vi "IVA Vision FPGA (Host).vi"() -> ()   [LabVIEW 2015]
uses:
  <vilib>/visionFPGA/Controls/IMAQ FPGA Image Size.ctl
  <vilib>/FPGAPlugInAG/cRIO-9030/niLvFpga_Open_cRIO-9030.vi
  <vilib>/rvi/interface/common/dynamic/niFpgaDynamicAddResources.vi
  <vilib>/FPGAPlugInAG/Dynamic/niLvFpga_Download_Dynamic.vi
  <vilib>/FPGAPlugInAG/Dynamic/niLvFpga_Run_Dynamic.vi
  <vilib>/visionFPGA/Basics/Configure Image Transfer from Target/IMAQ FPGA Configure Image Transfer from Target U8.vi
  <vilib>/visionFPGA/Basics/Image Transfer from Target/IMAQ FPGA Image Transfer from Target U8.vi
  <vilib>/visionFPGA/Basics/Configure Image Transfer to Target/IMAQ FPGA Configure Image Transfer to Target U32.vi
  <vilib>/visionFPGA/Basics/Image Transfer to Target/IMAQ FPGA Image Transfer to Target U32.vi
  <vilib>/FPGAPlugInAG/Dynamic/niLvFpga_Close_Dynamic.vi
  <vilib>/rvi/interface/nirviOpenFPGA/nirviOpenFPGA.xnode
  FPGA Bitfiles/IVAVisionFPGA.lvbitx
  IVA Vision FPGA (FPGA).vi
  <vilib>/rvi/interface/nirviMethod/nirviMethod.xnode
  <vilib>/rvi/interface/nirviCloseFPGA/nirviCloseFPGA.xnode
  <vilib>/visionFPGA/NI_VDM_FPGA_Basics.lvlib
panel:
  out "Image Out":T1(plugin-control)
  out "Error Out":errorcluster
  out "Image":T1(plugin-control)
  in  "Stop":bool
  in  "Image File Path":path
  # "Overview: Demonstrates how to use IMAQ FPGA Image Transfer Host to Target to transfer an image to a FPGA target for processing.\nRequirements:\n- LabVIEW FPGA\n- Vision Development Software\nInstructions:\n1. Select an Image File Path\n2. Run the VI."
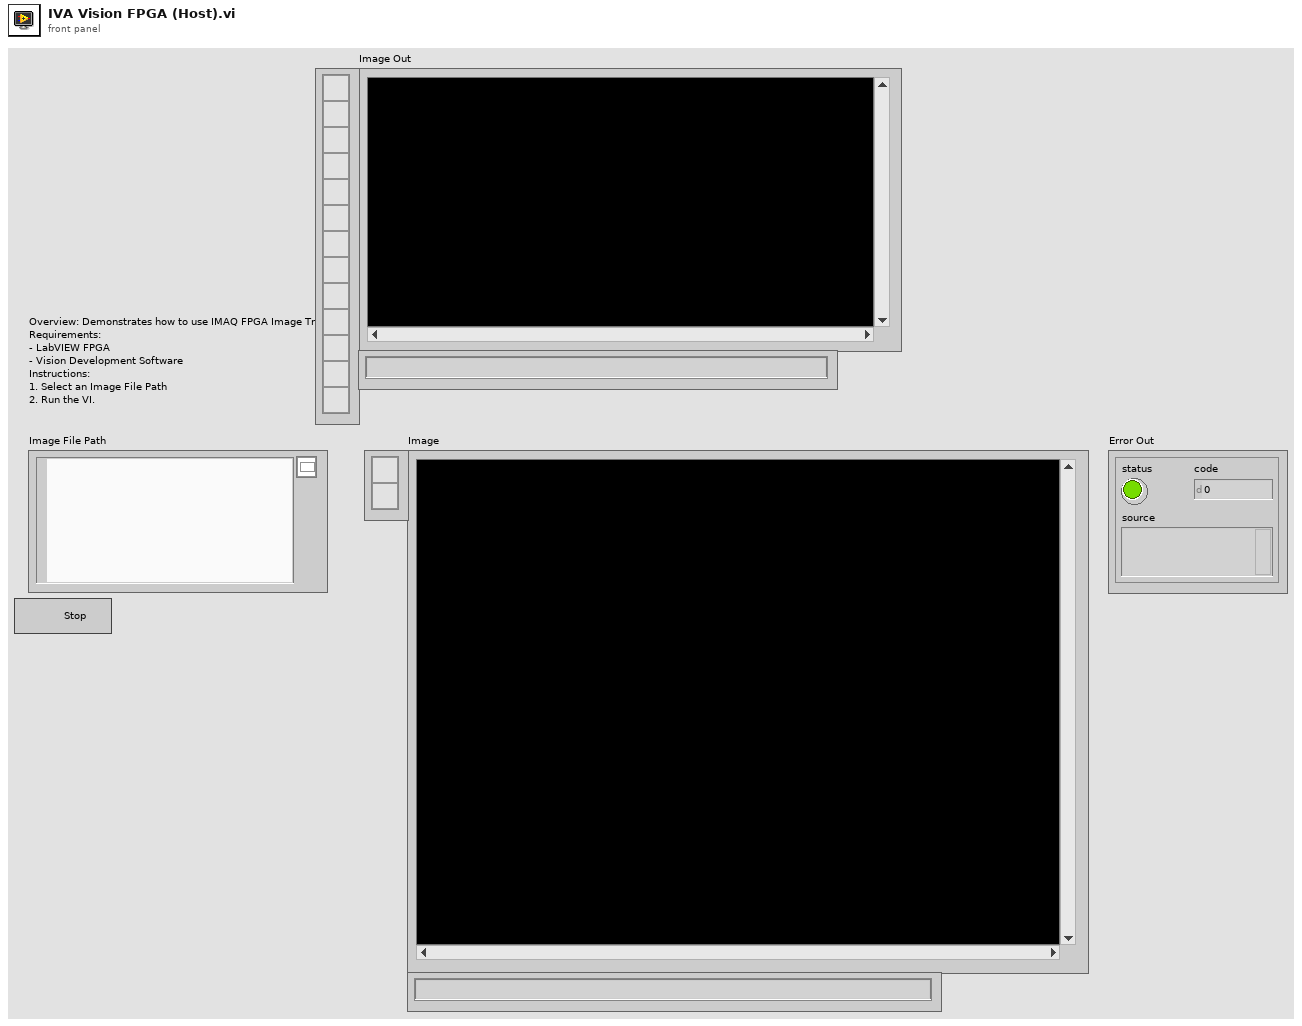
[diagram p1: front panel]
types:
  T1 = typedef "IMAQ Image.ctl" = refnum<image>
  T2 = typedef "IMAQ FPGA Image Size.ctl" = cluster{"Width":u32, "Height":u32}
  T3 = typedef "Image Type" = u32
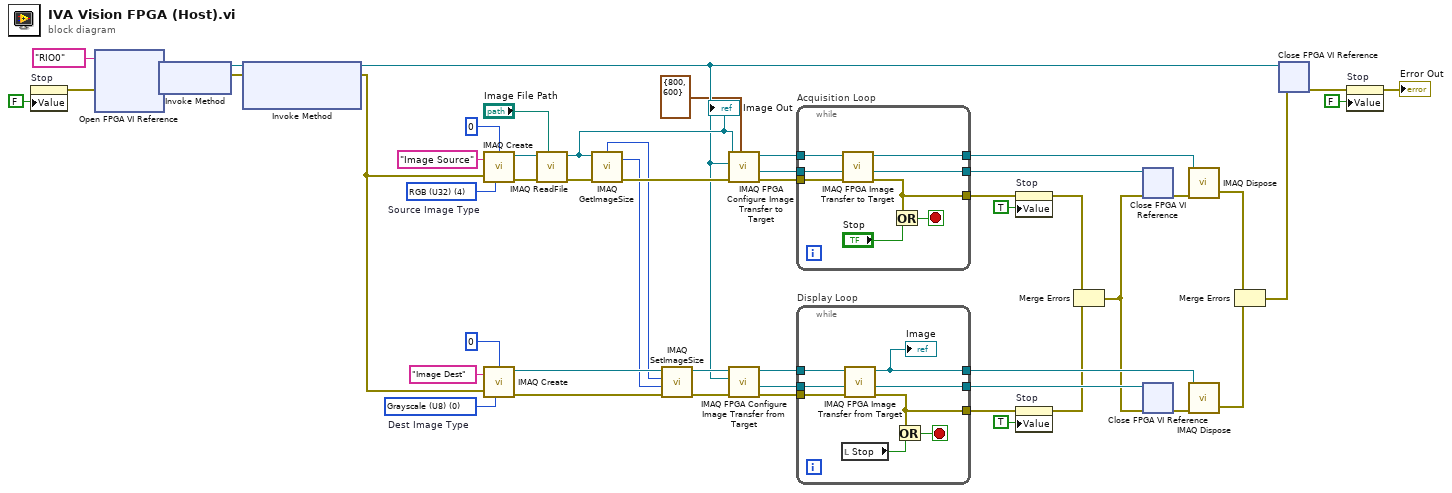
[diagram p0: block diagram]
diagram:
  w16 = T3 0 items=["Grayscale (U8)", "Grayscale (I16)", "Grayscale (SGL)", "Complex (CSG)", "RGB (U32)", "HSL (U32)", "RGB (U64)", "Grayscale (U16)"]  # Dest Image Type
  w17 = T3 4 items=["Grayscale (U8)", "Grayscale (I16)", "Grayscale (SGL)", "Complex (CSG)", "RGB (U32)", "HSL (U32)", "RGB (U64)", "Grayscale (U16)"]  # Source Image Type
  n1 = property on="Stop" class="Bool (strict)"("Value"=FALSE ("Stop")) -> (error out=w44:errorcluster)  [unwired: 2 in, 1 out]
  n2 = xnode "Open FPGA VI Reference"("error in"=w44, "resource name"=tag "RIO0") -> ("FPGA VI Reference Out"=w39:refnum<k20>, "error out"=w41:errorcluster)
  n3 = xnode "Invoke Method"("FPGA VI Reference In"=w39, "error in"=w41) -> ("FPGA VI Reference Out"=w43:refnum<k20>, "error out"=w42:errorcluster)
  n4 = xnode "Invoke Method"("FPGA VI Reference In"=w43, "error in"=w42) -> ("FPGA VI Reference Out"=w13:refnum<k20>, "error out"=w40:errorcluster)  [unwired: 1 in]
  n5 = call "IMAQ Create"("Border Size"=0, "Image Name"="Image Source", "Image Type"=w17, "error in (no error)"=w40) -> ("New Image"=w52:T1, "error out"=w51:errorcluster)  [unwired: 1 in]
  n6 = call "IMAQ Create"("Border Size"=0, "Image Name"="Image Dest", "Image Type"=w16, "error in (no error)"=w40) -> ("New Image"=w46:T1, "error out"=w14:errorcluster)  [unwired: 1 in]
  n7 = call "IMAQ ReadFile"("File Path"="Image File Path", "error in (no error)"=w51, "Image"=w52) -> ("error out"=w47:errorcluster, "Image Out"=w37:T1)  [unwired: 4 in, 3 out]
  "Image Out" <- w37
  n8 = call "IMAQ GetImageSize"("Image"=w37, "error in (no error)"=w47) -> ("Y Resolution"=w21:i32, "X Resolution"=w20:i32, "error out"=w38:errorcluster)  [unwired: 2 in]
  n9 = call "IMAQ SetImageSize"("error in (no error)"=w14, "Y Resolution"=w21, "X Resolution"=w20, "Image"=w46) -> ("error out"=w32:errorcluster, "Image Out"=w33:T1)  [unwired: 1 in]
  n10 = call-poly <vilib>:"IMAQ FPGA Configure Image Transfer to Target.vi"("Image Size"=T2 {"Width"=800, "Height"=600}, "error in (no error)"=w38, "FPGA VI Reference In"=w13, "Image"=w37) -> ("error out"=w34:errorcluster, "DMA FIFO Reference Out"=w35:refnum<k20>, "Image Out"=w36:T1)  [unwired: 4 in, 1 out]
  n11 = call-poly <vilib>:"IMAQ FPGA Configure Image Transfer from Target.vi"("error in (no error)"=w32, "FPGA VI Reference In"=w13, "Image"=w33) -> ("error out"=w30:errorcluster, "DMA FIFO Reference Out"=w29:refnum<k20>, "Image Out"=w31:T1)  [unwired: 6 in]
  n12 = while "Acquisition Loop" {
    tunnel: [w54] -> w12
    tunnel: w36 -> [w59]
    tunnel: w35 -> [w58]
    tunnel: w34 -> [w57]
    tunnel: [w56] -> w6
    tunnel: [w55] -> w28
    stop <- w60 stop-if-true
    n13 = call-poly <vilib>:"IMAQ FPGA Image Transfer to Target.vi"("error in (no error)"=w57, "DMA FIFO Reference In"=w58, "Image"=w59) -> ("error out"=w54:errorcluster, "DMA FIFO Reference Out"=w56:refnum<k20>, "Image Out"=w55:T1)  [unwired: 6 in]
    n14 = Or(x=w54, y="Stop") -> (x .or. y?=w60:bool)
  }
  n15 = while "Display Loop" {
    tunnel: w31 -> [w68]
    tunnel: [w66] -> w25
    tunnel: w30 -> [w65]
    tunnel: w29 -> [w64]
    tunnel: [w63] -> w26
    tunnel: [w62] -> w9
    stop <- w69 stop-if-true
    n16 = local read "Stop"() -> (w67:bool)
    n17 = call-poly <vilib>:"IMAQ FPGA Image Transfer from Target.vi"("error in (no error)"=w65, "DMA FIFO Reference In"=w64, "Image"=w68) -> ("error out"=w62:errorcluster, "DMA FIFO Reference Out"=w63:refnum<k20>, "Image Out"=w66:T1)  [unwired: 6 in]
    "Image" <- w66
    n18 = Or(x=w62, y=w67) -> (x .or. y?=w69:bool)
  }
  n19 = property on="Stop" class="Bool (strict)"(error in=w12, "Value"=TRUE ("Stop")) -> (error out=w8:errorcluster)  [unwired: 1 in, 1 out]
  n20 = property on="Stop" class="Bool (strict)"(error in=w9, "Value"=TRUE ("Stop")) -> (error out=w7:errorcluster)  [unwired: 1 in, 1 out]
  n21 = Merge Errors(w8, w7) -> (w5:errorcluster)
  n22 = xnode "Close FPGA VI Reference"("FPGA VI Reference In"=w6, "error in"=w5) -> ("error out"=w27:errorcluster)
  n23 = xnode "Close FPGA VI Reference"("FPGA VI Reference In"=w26, "error in"=w5) -> ("error out"=w24:errorcluster)
  n24 = call "IMAQ Dispose"("Image"=w28, "error in (no error)"=w27) -> ("error out"=w22:errorcluster)  [unwired: 4 in]
  n25 = call "IMAQ Dispose"("Image"=w25, "error in (no error)"=w24) -> ("error out"=w23:errorcluster)  [unwired: 4 in]
  n26 = Merge Errors(w22, w23) -> (w15:errorcluster)
  n27 = xnode "Close FPGA VI Reference"("FPGA VI Reference In"=w13, "error in"=w15) -> ("error out"=w3:errorcluster)
  n28 = property on="Stop" class="Bool (strict)"(error in=w3, "Value"=FALSE ("Stop")) -> (error out=→"Error Out":errorcluster)  [unwired: 1 in, 1 out]
